vi "Extract from Tree Tag.vi"(11 "Tag":string) -> (2 "WID":string, 3 "DC_UID":T1)   [LabVIEW 2017, in "Application Manager.lvclass"]
doc: "Extract the Debug Client UID and the Worker ID from the Tag"
uses:
  Application Manager.lvclass
  Common VIs/DC_UID.ctl
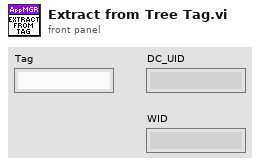
[diagram p1: front panel]
types:
  T1 = typedef "DC_UID.ctl" = string
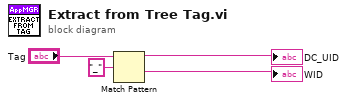
[diagram p0: block diagram]
diagram:
  n1 = Match Pattern(string="Tag", regular expression="_") -> (before substring=→"DC_UID":string, after substring=→"WID":string)  [unwired: 1 in, 2 out]
